vi "relative_error_fgv.vi"(8 "Error In":errorcluster, 9 "Knob":dbl, 10 "Amp String":string, 11 "Action":T1) -> (0 "Error Out":errorcluster, 1 "Error String":string, 2 "Incremented String":string, 3 "Starting String":string, 5 "Indicator String":string)   [LabVIEW 2021, in "Signal.lvlib"]
doc: "This FGV is used to memorize the realtive error."
uses:
  Signal.lvlib
  Tipski Definicii/rel_error.ctl
  Tipski Definicii/Signal Values.ctl
  Tipski Definicii/Unit.ctl
panel:
  # "Input"
  # "Output"
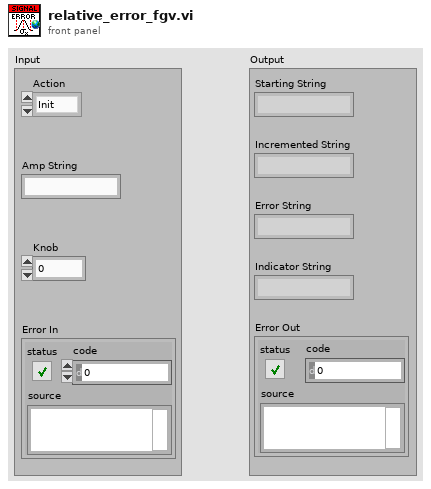
[diagram p1: front panel]
types:
  T1 = typedef "rel_error.ctl" = enum16{"Init", "Add String", "Error", "Get Error and Strings", "Reset"}
  T2 = typedef "Unit.ctl" = enum16{"Init", "Add", "Read"}
  T3 = typedef "Signal Values.ctl" = enum16{"Init", "Add V/A string", "Add Hz string", "Get Strings and Values", "Reset", "Add Offset", "Add Waveform", "Add Phase"}
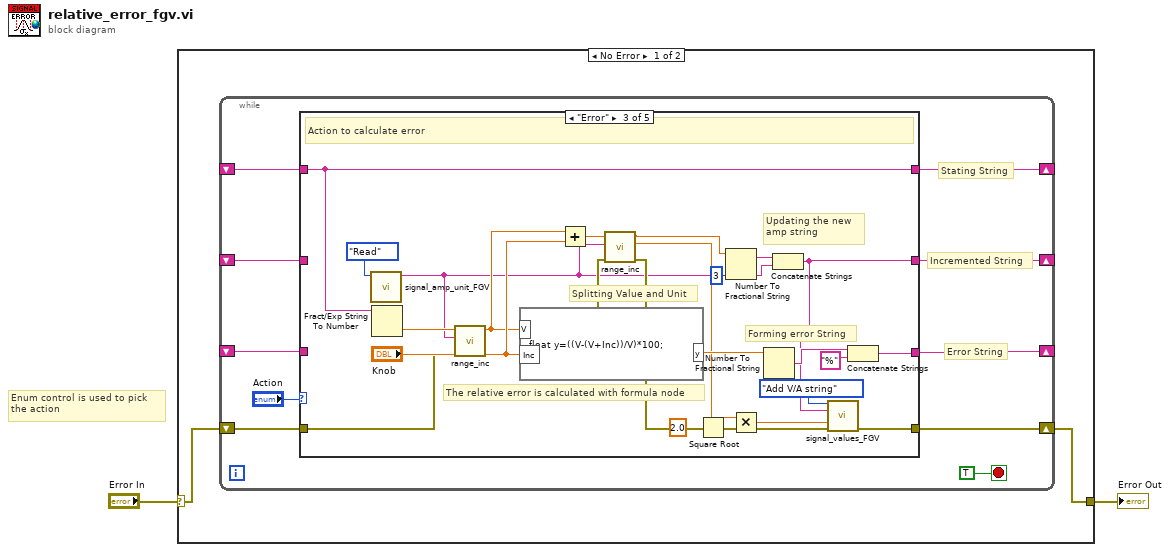
[diagram p0: block diagram]
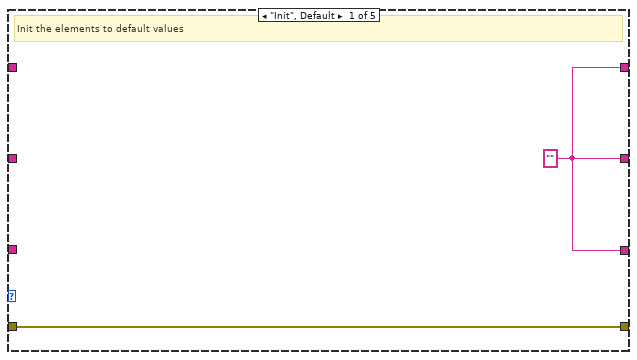
[diagram p2: hidden frame]
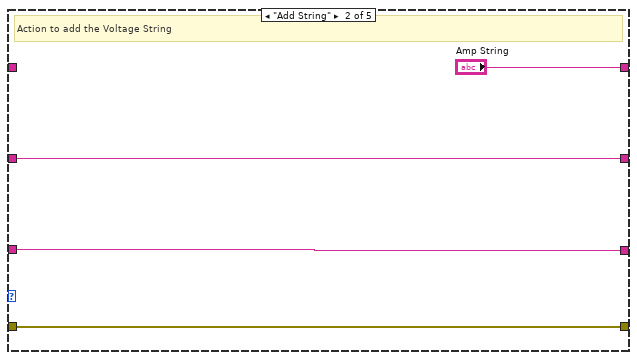
[diagram p3: hidden frame]
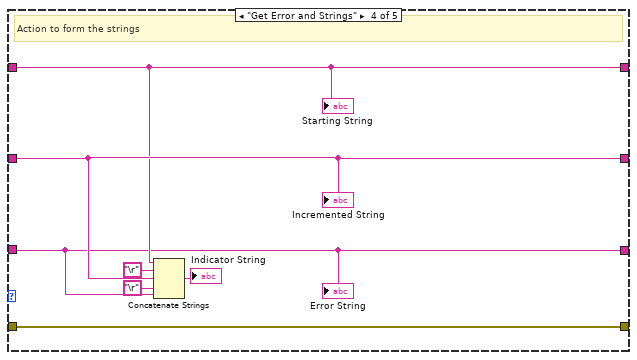
[diagram p4: hidden frame]
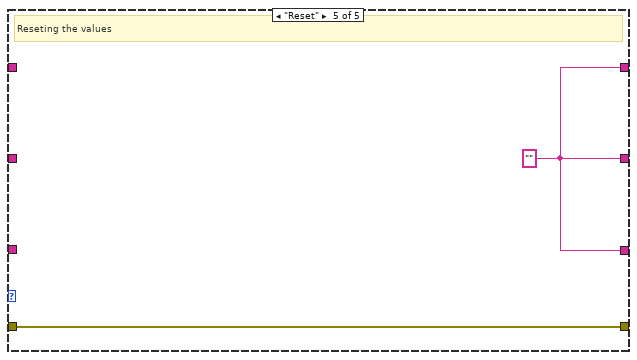
[diagram p5: hidden frame]
diagram:
  # "Enum control is used to pick \nthe action"
  n1 = case shown="No Error" "Error In" {
    selector: "Error In" -> [w4 w54]
    tunnel: [w3 w54] -> w1
    frame No Error {
      n2 = while {
        shift-right: [w10] -> _
        shift-left: _ -> [w9]
        shift-right: [w11] -> _
        shift-left: _ -> [w8]
        shift-right: [w12] -> _
        shift-left: _ -> [w7]
        shift-right: [w5] -> w3
        shift-left: w4 -> [w6]
        stop <- TRUE stop-if-true
        # "Incremented String"
        # "Error String"
        # "Stating String"
        n3 = case shown="\"Error\"" "Action" {
          tunnel: [w16 w20 w41 w47 w52] -> w12
          tunnel: [w16 w18 w35 w49 w52] -> w11
          tunnel: [w16 "Amp String" w39 w48 w52] -> w10
          tunnel: w9 -> [_ _ w39 w48 _]
          tunnel: w8 -> [_ w18 _ w49 _]
          tunnel: w7 -> [_ w20 _ w47 _]
          tunnel: w6 -> [w15 w17 w29 w45 w53]
          tunnel: [w15 w17 w38 w45 w53] -> w5
          frame "Init", Default {
            w16 = ""
            # "Init the elements to default values"
          }
          frame "Add String" {
            # "Action to add the Voltage String"
          }
          frame "Error" {
            # "Forming error String"
            # "Updating the new \namp string"
            # "Splitting Value and Unit"
            # "The relative error is calculated with formula node"
            # "Action to calculate error"
            n4 = call "signal_amp_unit_FGV.vi"("Action"=Unit."Read") -> ("Unit (Not F)"=w25:string)  [unwired: 8 in, 2 out]
            n5 = Fract/Exp String To Number(string=w39) -> (number=w31:dbl)  [unwired: 3 in, 1 out]
            n6 = call "range_inc.vi"("Error In"=w29, "Unit"=w25, "Amp"=w31) -> ("Error Out"=w28:errorcluster, "Amp String"=w30:dbl)  [unwired: 6 in, 1 out]
            n7 = formula code="float y=((V-(V+Inc))/V)*100;"("Inc"="Knob", "V"=w30) -> ("y"=w44:dbl)
            n8 = Add(x=w30, y="Knob") -> (x+y=w33:dbl)
            n9 = call "range_inc.vi"("Error In"=w28, "Unit"=w25, "Amp"=w33) -> ("Error Out"=w27:errorcluster, "Amp Base"=w24:dbl, "Amp String"=w32:dbl)  [unwired: 6 in]
            n10 = Square Root(x=2.0) -> (sqrt(x)=w22:dbl)
            n11 = Number To Fractional String(number=w32, precision (6)=i16 3) -> (F-format string=w37:string)  [unwired: 2 in]
            n12 = Multiply(x=w24, y=w22) -> (x*y=w23:dbl)
            n13 = Number To Fractional String(number=w44) -> (F-format string=w43:string)  [unwired: 3 in]
            n14 = Concatenate Strings(w37, w25) -> (w35:string)
            n15 = call "signal_values_FGV.vi"("Action"=Signal_Values."Add V/A string", "Amp String"=w35, "Amp Value"=w23, "Error In"=w27) -> ("Error Out"=w38:errorcluster)  [unwired: 10 in, 1 out]
            n16 = Concatenate Strings(w43, "%" ("string")) -> (w41:string)
          }
          frame "Get Error and Strings" {
            # "Action to form the strings"
            n17 = Concatenate Strings(w48, "\r", w49, "\r", w47) -> (→"Indicator String":string)
            "Starting String" <- w48
            "Incremented String" <- w49
            "Error String" <- w47
          }
          frame "Reset" {
            w52 = ""
            # "Reseting the values"
          }
        }
      }
    }
    frame Error {
    }
  }
  "Error Out" <- w1
